vi "midiOutClose.vi"(8 "error in":errorcluster, 11 "midi in":refnum<class "midi.lvclass">) -> (0 "error out":errorcluster, 3 "midi out":refnum<class "midi.lvclass">)   [LabVIEW 2020, in "midi.lvclass"]
doc: "The midiOutClose function closes the specified MIDI output device."
uses:
  midi.lvclass
  midi.lvclass/midi.ctl
  winmm.dll
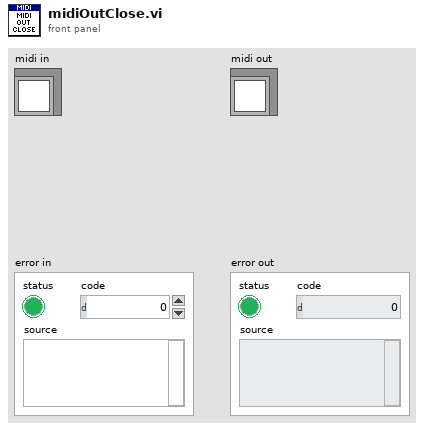
[diagram p1: front panel]
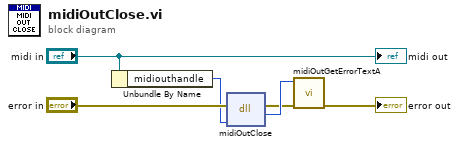
[diagram p0: block diagram]
diagram:
  n1 = Unbundle By Name("midi in") -> ("midiouthandle"=w1:u64)
  n2 = dll-call lib="winmm.dll" fn="midiOutClose"(error in="error in", "hmidiout"=w1) -> (error out=w2:errorcluster, "return type"=w6:i32)  [unwired: 3 in, 1 out]
  n3 = call "midiOutGetErrorTextA.vi"("error in"=w2, "Error Code"=w6) -> ("error out"=→"error out":errorcluster)  [unwired: 9 in]
  "midi out" <- "midi in"
